vi "Save.vi"(8 "error in (no error)":errorcluster, 11 "Vision in":refnum<class "Vision.lvclass">) -> (0 "error out":errorcluster, 3 "Vision out":refnum<class "Vision.lvclass">)   [LabVIEW 2019, in "Vision.lvlib" / "Vision.lvclass"]
uses:
  Vision.lvclass
  Vision.lvclass/Vision.ctl
  e9838fd0-2cc1-44de-be83-0f9f541addb3.vi
  7dcd0526-b95c-47ac-8e4b-7d5e9dfb3bc2.vi
  <vilib>/JDP Science/JSONtext/Variant to JSON Text.vi
  <vilib>/JDP Science/JSONtext/LVClass Serializer/JSONtext LVClass Serializer.lvclass
  <vilib>/JDP Science/JSONtext/JSONtext.lvlib
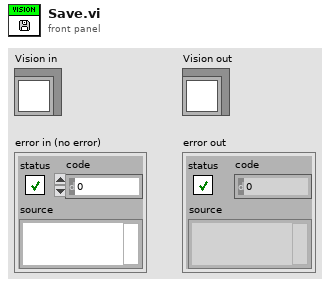
[diagram p1: front panel]
types:
  T1 = typedef "IMAQdx.ctl" = refnum<k21>
  T2 = cluster{"Global Rectangle":i32[], "Contours":cluster{"Contour Type":u32, "ROI Type":u32, "Points":i32[]}[]}
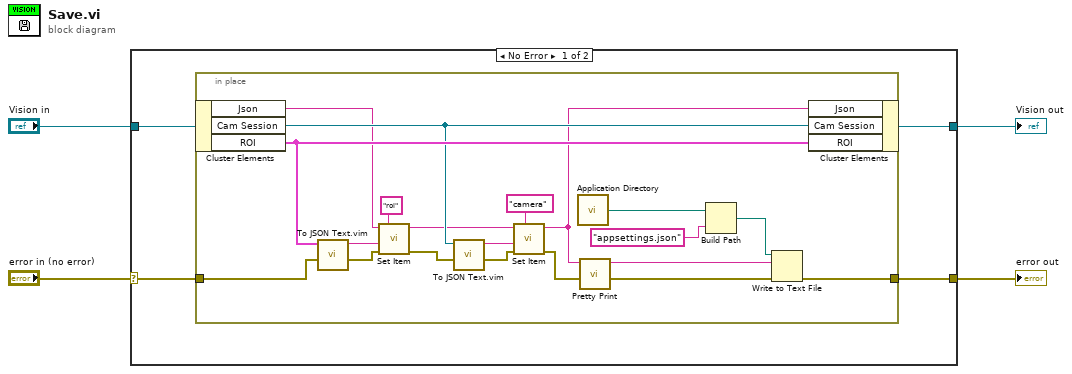
[diagram p0: block diagram]
diagram:
  n1 = case shown="No Error" "error in (no error)" {
    selector: "error in (no error)" -> [w6 w29]
    tunnel: [w5 w29] -> w3
    tunnel: [w7 w28] -> w1
    tunnel: "Vision in" -> [w8 w28]
    frame No Error {
      n2 = in-place {
        in-place-border: w6 -> [w25]
        in-place-border: [w11] -> w5
        n3 = in-place-cluster #1(w8) -> ("Json"=w16:string, "Cam Session"=w22:T1, "ROI"=w27:T2)
        n4 = call "To JSON Text.vim"("error in (no error)"=w25, "Anything"=w27) -> ("error out"=w23:errorcluster, "<JSON>"=w26:string)  [unwired: 8 in]
        n5 = call <vilib>:"Set Item.vi"("$Path or Item Name"="roi", "error in (no error)"=w23, "JSON to Insert"=w26, "JSON"=w16) -> ("error out"=w19:errorcluster, "<JSON>"=w21:string)  [unwired: 4 in, 1 out]
        n6 = call "To JSON Text.vim"("error in (no error)"=w19, "Anything"=w22) -> ("error out"=w18:errorcluster, "<JSON>"=w20:string)  [unwired: 8 in]
        n7 = call <vilib>:"Set Item.vi"("$Path or Item Name"="camera", "error in (no error)"=w18, "JSON to Insert"=w20, "JSON"=w21) -> ("error out"=w12:errorcluster, "<JSON>"=w10:string)  [unwired: 4 in, 1 out]
        n8 = call <vilib>:"Application Directory.vi"() -> ("Application Directory"=w15:path)
        n9 = call <vilib>:"Pretty Print.vi"("JSON"=w10) -> ("<JSON>"=w9:string)  [unwired: 8 in, 2 out]
        n10 = Build Path(base path=w15, name or relative path="appsettings.json") -> (appended path=w13:path)
        n11 = Write to Text File(file (use dialog)=w13, text=w9, error in=w12) -> (error out=w11:errorcluster)  [unwired: 1 in, 2 out]
        n12 = in-place-cluster #1("Json"=w10, "Cam Session"=w22, "ROI"=w27) -> (w7:refnum<class "Vision.lvclass">)
      }
    }
    frame Error {
    }
  }
  "error out" <- w3
  "Vision out" <- w1
